vi "Transmit Configuration Data's.vi"(7 "Data Cluster In":T1, 8 "error in (no error)":errorcluster) -> (0 "error out":errorcluster, 5 "Data Cluster Out":T1)   [LabVIEW 2021, in "Test Configuration.lvlib"]
doc: "<b>Note:</b> This VI was modified by the <b>Validate DQMH Module</b> tool to turn off automatic error handling."
uses:
  Test Configuration.lvlib
  Module Data--cluster.ctl
  <vilib>/addons/_JKI.lib/Serialization/JSON/Library/Flatten To JSON String.vi
  RT Acquisition Engine/RT Acquisition Engine.lvlib
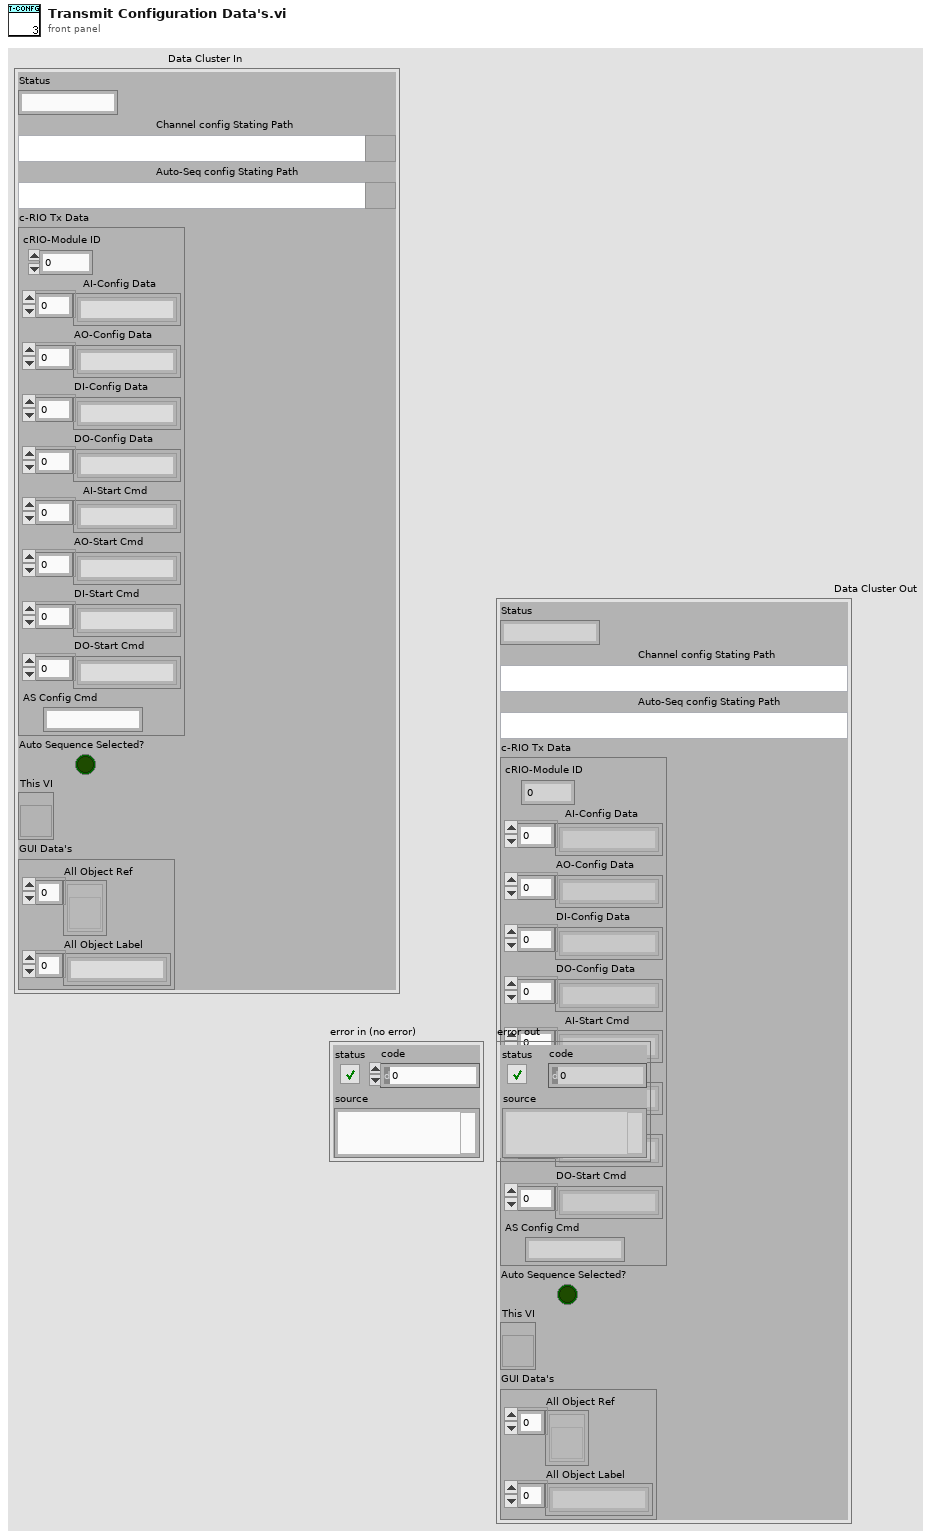
[diagram p1: front panel]
types:
  T1 = typedef "Test Configuration.lvlib/Module Data--cluster.ctl" = cluster{"Status":string, "Channel config Stating Path":path, "Auto-Seq config Stating Path":path, "c-RIO Tx Data":cluster{"cRIO-Module ID":i32, "AI-Config Data":string[], "AO-Config Data":string[], "DI-Config Data":string[], "DO-Config Data":string[], "AI-Start Cmd":string[], "AO-Start Cmd":string[], "DI-Start Cmd":string[], "DO-Start Cmd":string[], "AS Config Cmd":string}, "Auto Sequence Selected?":bool, "This VI":refnum<vi>, "GUI Data's":cluster{"All Object Ref":refnum<vi>[], "All Object Label":string[]}}
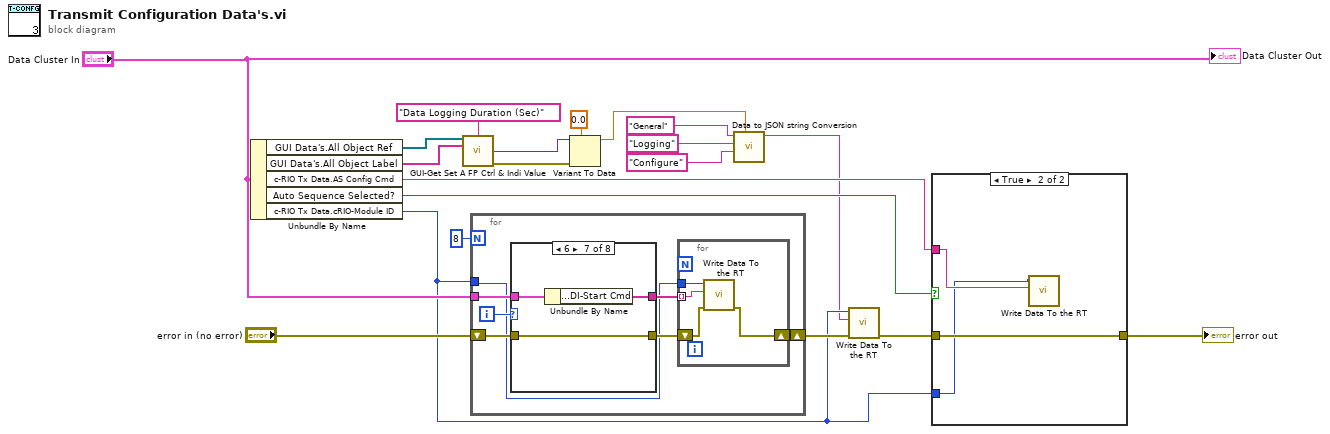
[diagram p0: block diagram]
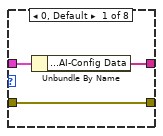
[diagram p3: hidden frame]
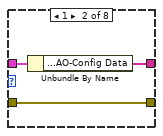
[diagram p4: hidden frame]
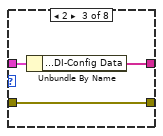
[diagram p5: hidden frame]
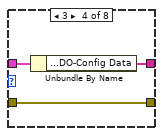
[diagram p6: hidden frame]
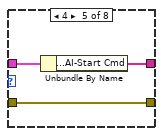
[diagram p7: hidden frame]
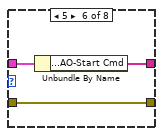
[diagram p8: hidden frame]
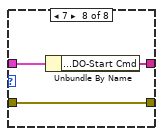
[diagram p9: hidden frame]
diagram:
  n1 = Unbundle By Name("Data Cluster In") -> ("GUI Data's.All Object Ref"=w11:refnum<vi>[], "GUI Data's.All Object Label"=w10:string[], "c-RIO Tx Data.AS Config Cmd"=w15:string, "Auto Sequence Selected?"=w17:bool, "c-RIO Tx Data.cRIO-Module ID"=w12:i32)
  n2 = call "GUI-Get Set A FP Ctrl & Indi Value.vi"("All Object Ref"=w11, "Label"="Data Logging Duration (Sec)", "All Object Label"=w10) -> ("Ctrl Value Out"=w7:variant, "error out"=w8:errorcluster)  [unwired: 9 in, 2 out]
  n3 = for {
    N: 8 -> [_]
    tunnel: "Data Cluster In" -> [w26]
    tunnel: w12 -> [w21]
    shift-right: [w23] -> w14
    shift-left: "error in (no error)" -> [w25]
    i -> [w27]
    n4 = case shown="6" w27 {
      tunnel: w26 -> [w34 w36 w39 w42 w45 w48 w51 w54]
      tunnel: w25 -> [w32 w37 w40 w43 w46 w49 w52 w55]
      tunnel: [w32 w37 w40 w43 w46 w49 w52 w55] -> w24
      tunnel: [w33 w35 w38 w41 w44 w47 w50 w53] -> w22
      frame 0, Default {
        n5 = Unbundle By Name(w34) -> ("c-RIO Tx Data.AI-Config Data"=w33:string[])
      }
      frame 1 {
        n6 = Unbundle By Name(w36) -> ("c-RIO Tx Data.AO-Config Data"=w35:string[])
      }
      frame 2 {
        n7 = Unbundle By Name(w39) -> ("c-RIO Tx Data.DI-Config Data"=w38:string[])
      }
      frame 3 {
        n8 = Unbundle By Name(w42) -> ("c-RIO Tx Data.DO-Config Data"=w41:string[])
      }
      frame 4 {
        n9 = Unbundle By Name(w45) -> ("c-RIO Tx Data.AI-Start Cmd"=w44:string[])
      }
      frame 5 {
        n10 = Unbundle By Name(w48) -> ("c-RIO Tx Data.AO-Start Cmd"=w47:string[])
      }
      frame 6 {
        n11 = Unbundle By Name(w51) -> ("c-RIO Tx Data.DI-Start Cmd"=w50:string[])
      }
      frame 7 {
        n12 = Unbundle By Name(w54) -> ("c-RIO Tx Data.DO-Start Cmd"=w53:string[])
      }
    }
    n13 = for {
      shift-right: [w30] -> w23
      shift-left: w24 -> [w31]
      tunnel: w22 -> [w29] mode=indexing
      tunnel: w21 -> [w28]
      n14 = call "Write Data To the RT.vi"("error in"=w31, "Data In"=w29, "Module ID"=w28) -> ("error out"=w30:errorcluster)  [unwired: 8 in]
    }
  }
  n15 = Variant To Data(error in=w8, type=0.0, Variant=w7) -> (data=w2:dbl)  [unwired: 1 out]
  n16 = call "Data to JSON string Conversion.vi"("Data"=w2, "SubCmd"="Configure", "Command"="Logging", "Interface"="General") -> ("Cmd String"=w1:string)  [unwired: 6 in, 1 out]
  n17 = call "Write Data To the RT.vi"("error in"=w14, "Data In"=w1, "Module ID"=w12) -> ("error out"=w13:errorcluster)  [unwired: 8 in]
  n18 = case shown="True" w17 {
    tunnel: w13 -> [w56 w59]
    tunnel: [w56 w59] -> w16
    tunnel: w15 -> [_ w58]
    tunnel: w12 -> [_ w57]
    frame False {
    }
    frame True {
      n19 = call "Write Data To the RT.vi"("Data In"=w58, "Module ID"=w57) -> ()  [unwired: 9 in, 1 out]
    }
  }
  "error out" <- w16
  "Data Cluster Out" <- "Data Cluster In"
